vi "COMMAND_GetCurrentPosition.vi"(8 "error in (no error)":errorcluster, 11 "StageDL090602SutterMP285 in":refnum<class "StageDL090602SutterMP285.lvclass">) -> (0 "error out":errorcluster, 2 "current position":refnum<class "SpaceVector.lvclass">, 3 "StageDL090602SutterMP285 out":refnum<class "StageDL090602SutterMP285.lvclass">)   [LabVIEW 2010, in "StageDL090602SutterMP285.lvclass"]
uses:
  StageDL090602SutterMP285.lvclass
  common/classes/SpaceVector/SpaceVector/SpaceVector.lvclass
  StageDL090602SutterMP285.lvclass/StageDL090602SutterMP285.ctl
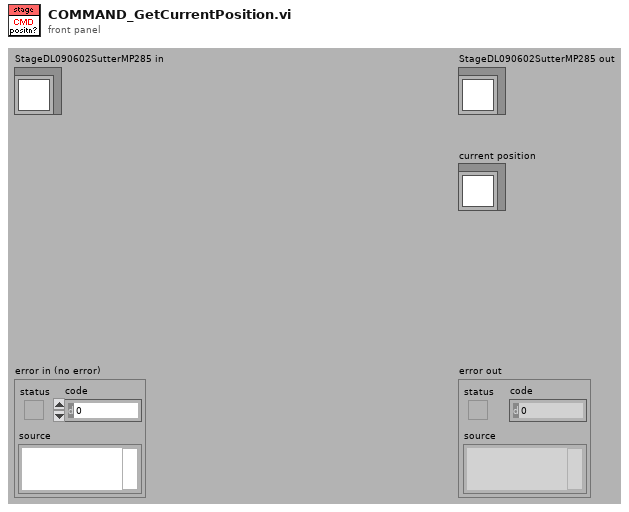
[diagram p1: front panel]
types:
  T1 = cluster{"[0]":dbl[unit], "[1]":dbl[unit], "[2]":dbl[unit]}
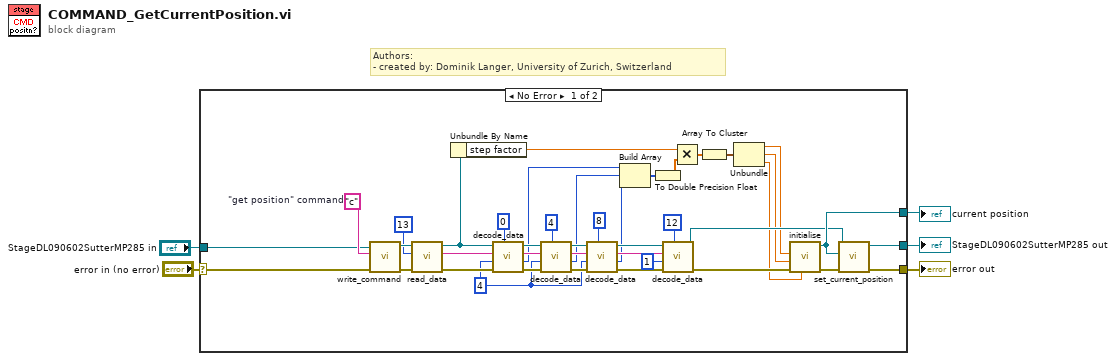
[diagram p0: block diagram]
diagram:
  # "Authors: \n- created by: Dominik Langer, University of Zurich, Switzerland"
  n1 = case shown="No Error" "error in (no error)" {
    selector: "error in (no error)" -> [w40 w48]
    tunnel: [w39 w48] -> w4
    tunnel: [w37 w47] -> w2
    tunnel: "StageDL090602SutterMP285 in" -> [w38 w47]
    tunnel: [w36 _] -> w1
    frame No Error {
      w24 = 4 ("length")
      w46 = "c"  # "get position" command
      n2 = call-dynamic "write_command.vi"("error in (no error)"=w40, "command (without terminating \"\\n\")"=w46, "DL090602SutterMP285Stage in"=w38) -> ("error out"=w45:errorcluster, "DL090602SutterMP285Stage out"=w44:refnum<class "StageDL090602SutterMP285.lvclass">)  [unwired: 7 out]
      n3 = call-dynamic "read_data.vi"("error in (no error)"=w45, "bytes to read"=u32 13, "DL090602SutterMP285Stage in"=w44) -> ("error out"=w42:errorcluster, "hex data string"=w41:string, "DL090602SutterMP285Stage out"=w7:refnum<class "StageDL090602SutterMP285.lvclass">)  [unwired: 6 out]
      n4 = Unbundle By Name(w7) -> ("step factor"=w6:dbl[unit])
      n5 = call-dynamic "decode_data.vi"("offset"=0, "error in (no error)"=w42, "length"=w24, "encoded data string in"=w41, "DL090602SutterMP285Stage in"=w7) -> ("error out"=w34:errorcluster, "decoded data"=w21:i32, "encoded data string out"=w32:string, "DL090602SutterMP285Stage out"=w33:refnum<class "StageDL090602SutterMP285.lvclass">)  [unwired: 3 out]
      n6 = call-dynamic "decode_data.vi"("offset"=4, "error in (no error)"=w34, "length"=w24, "encoded data string in"=w32, "DL090602SutterMP285Stage in"=w33) -> ("error out"=w30:errorcluster, "decoded data"=w19:i32, "encoded data string out"=w28:string, "DL090602SutterMP285Stage out"=w25:refnum<class "StageDL090602SutterMP285.lvclass">)  [unwired: 3 out]
      n7 = call-dynamic "decode_data.vi"("offset"=8, "error in (no error)"=w30, "length"=w24, "encoded data string in"=w28, "DL090602SutterMP285Stage in"=w25) -> ("error out"=w27:errorcluster, "decoded data"=w20:i32, "encoded data string out"=w23:string, "DL090602SutterMP285Stage out"=w26:refnum<class "StageDL090602SutterMP285.lvclass">)  [unwired: 3 out]
      n8 = Build Array(w21, w19, w20) -> (w22:i32[])
      n9 = To Double Precision Float(number=w22) -> (double precision float=w18:dbl[])
      n10 = call-dynamic "decode_data.vi"("offset"=12, "error in (no error)"=w27, "length"=1, "encoded data string in"=w23, "DL090602SutterMP285Stage in"=w26) -> ("error out"=w17:errorcluster, "DL090602SutterMP285Stage out"=w15:refnum<class "StageDL090602SutterMP285.lvclass">)  [unwired: 5 out]
      n11 = Multiply(x=w6, y=w18) -> (x*y=w14:dbl[unit][])
      n12 = Array To Cluster(array=w14) -> (cluster=w13:T1)
      n13 = Unbundle(w13) -> ("[0]"=w12:dbl[unit], "[1]"=w11:dbl[unit], "[2]"=w10:dbl[unit])
      n14 = call "initialise.vi"("z"=w10, "error in (no error)"=w17, "y"=w11, "x"=w12) -> ("error out"=w16:errorcluster, "SpaceVector out"=w36:refnum<class "SpaceVector.lvclass">)  [unwired: 6 out]
      n15 = call-dynamic "set_current_position.vi"("error in (no error)"=w16, "current position"=w36, "DL090409StageScaffold.lvclass in"=w15) -> ("error out"=w39:errorcluster, "DL090409StageScaffold.lvclass out"=w37:refnum<class "StageDL090602SutterMP285.lvclass">)  [unwired: 7 out]
    }
    frame Error {
    }
  }
  "error out" <- w4
  "StageDL090602SutterMP285 out" <- w2
  "current position" <- w1
